vi "frequancy translation for DSBSC (AM).vi"() -> ()   [LabVIEW 2018]
uses:
  <vilib>/express/express analysis/Spectral/Block/exnSpectralBlock spectral measurements RMS poly.vi
  <vilib>/express/express analysis/Spectral/Block/exnSpectralBlock spectral measurements RMS DDT.vi
  <vilib>/express/express analysis/Spectral/XNode/ExpressSpectralMeasurementsBlockNode.xnode
panel:
  out "SSB":dynamicdata(graph)
  out "Waveform Graph 5":dynamicdata(graph)
  out "Waveform Graph 3":dynamicdata(graph)
  out "Waveform Graph 4":dynamicdata(graph)
  out "Waveform Graph 2":dynamicdata(graph)
  in  "fm":dbl
  in  "fc":dbl
  in  "stop":bool
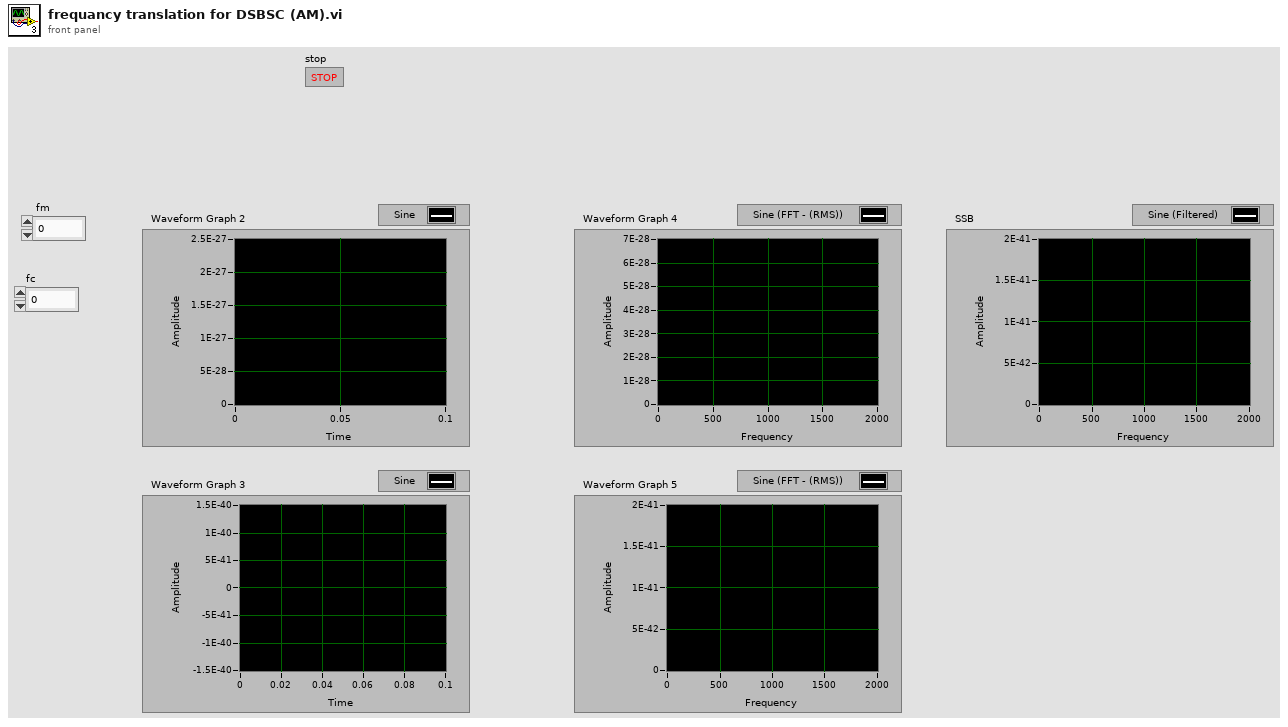
[diagram p1: front panel]
types:
  T1 = cluster{"averaging mode":u16, "weighting mode":u16, "number of averages":u32}
  T2 = cluster{"dB On (F)":bool, "unwrap phase (F)":bool, "convert to degree (F)":bool}
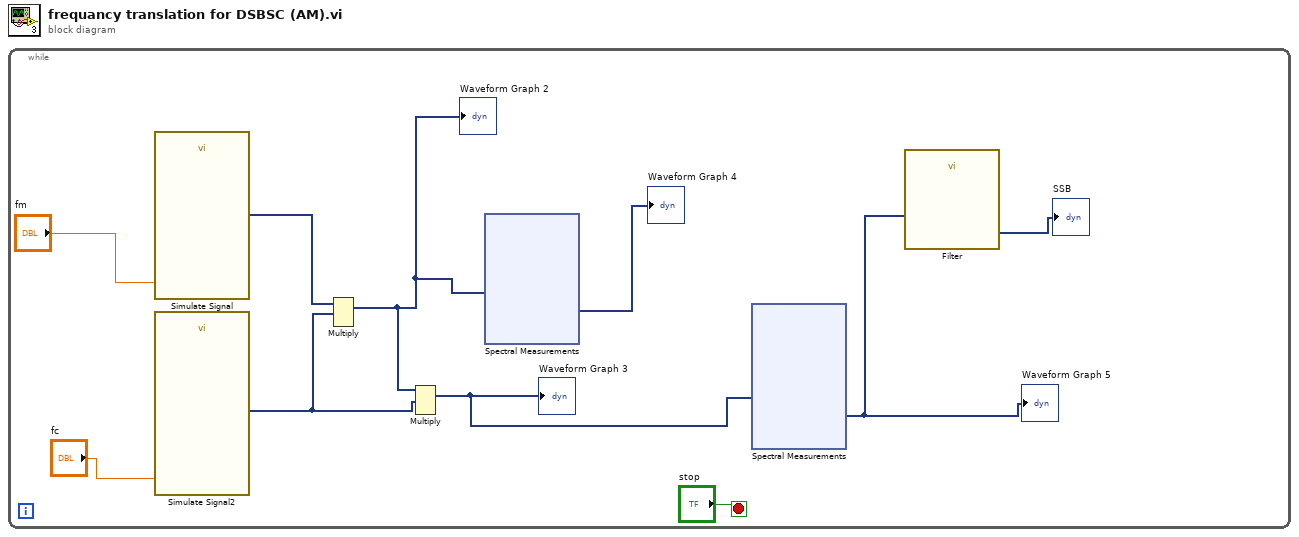
[diagram p0: block diagram]
diagram:
  n1 = while {
    stop <- "stop" stop-if-true
    n2 = call "Simulate Signal"("Frequency"="fm") -> ("Sine"=w7:dynamicdata)  [unwired: 13 in, 1 out]
    n3 = call "Simulate Signal2"("Frequency"="fc") -> ("Sine"=w4:dynamicdata)  [unwired: 13 in, 1 out]
    n4 = Multiply(1:w4, 2:w7) -> (0:w5:dynamicdata)  [unwired: 1 in, 1 out]
    "Waveform Graph 2" <- w5
    n5 = Multiply(1:w4, 2:w5) -> (0:w3:dynamicdata)  [unwired: 1 in, 1 out]
    "Waveform Graph 3" <- w3
    n6 = xnode "Spectral Measurements"("Signals"=w5) -> ("FFT - (RMS)"=→"Waveform Graph 4":dynamicdata)  [unwired: 1 in, 2 out]
    n7 = xnode "Spectral Measurements"("Signals"=w3) -> ("FFT - (RMS)"=w2:dynamicdata)  [unwired: 1 in, 2 out]
    "Waveform Graph 5" <- w2
    n8 = call "Filter"("Signal"=w2) -> ("Filtered Signal"=→"SSB":dynamicdata)  [unwired: 9 in, 1 out]
  }
